vi "5492_Zero Yaw.vi"(7 "Device Number":T1, 8 "error in":errorcluster, 10 "Zero":bool) -> (0 "error out":errorcluster)   [LabVIEW 2016]
uses:
  <vilib>/Rock Robotics/WPI/ThirdParty/Sensors/navX/_TypeDefs/FRIC_navX_DeviceNumbersTypeDef.ctl
  <vilib>/Rock Robotics/WPI/ThirdParty/Sensors/navX/_TypeDefs/Z900_navX_ActionTypeDef.ctl
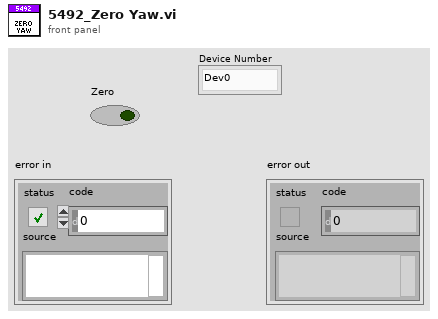
[diagram p1: front panel]
types:
  T1 = typedef "FRIC_navX_DeviceNumbersTypeDef.ctl" = enum16{"Dev0", "Dev1", "Dev2", "Dev3"}
  T2 = typedef "Z900_navX_ActionTypeDef.ctl" = enum16{"None", "Halt", "Normal Read", "Update Serial Protocol", "Update Rate Htz", "Zero-Yaw", "Zero-Displacement", "Zero-Velocity"}
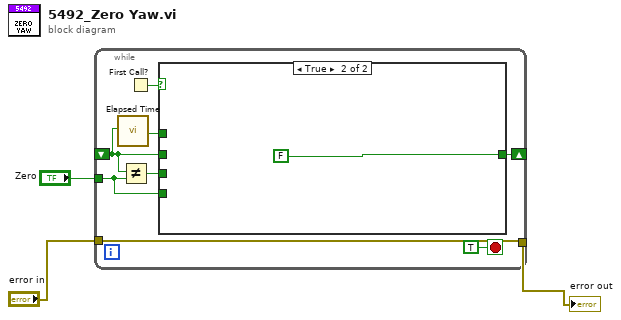
[diagram p0: block diagram]
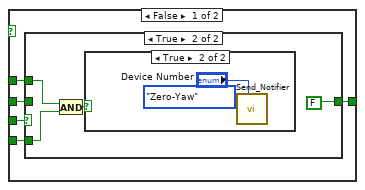
[diagram p2: hidden frame]
diagram:
  n1 = while {
    shift-right: [w10] -> _
    shift-left: _ -> [w5]
    tunnel: "Zero" -> [w7]
    tunnel: [w4] -> w2
    tunnel: "error in" -> [w4]
    stop <- TRUE stop-if-true
    n2 = call "Elapsed Time"("Reset"=w5) -> ("Time has Elapsed"=w6:bool)  [unwired: 11 in, 7 out]
    n3 = Not Equal?(x=w5, y=w7) -> (x != y?=w9:bool)
    n4 = First Call?() -> (First Call?: T/F=w8:bool)
    n5 = case shown="True" w8 {
      tunnel: [w16 FALSE] -> w10
      tunnel: w5 -> [w15 _]
      tunnel: w9 -> [w14 _]
      tunnel: w7 -> [w13 _]
      tunnel: w6 -> [w12 _]
      frame False {
        n6 = case shown="True" w14 {
          tunnel: [w17 FALSE] -> w16
          tunnel: w15 -> [w17 _]
          tunnel: w13 -> [_ w21]
          tunnel: w12 -> [_ w19]
          frame False {
          }
          frame True {
            n7 = And(x=w19, y=w21) -> (x .and. y?=w20:bool)
            n8 = case shown="True" w20 {
              frame False {
              }
              frame True {
                n9 = call <vilib>:"Send_Notifier.vi"("Device Number"="Device Number", "navX Action"=Z900_navX_ActionTypeDef."Zero-Yaw") -> ()  [unwired: 10 in]
              }
            }
          }
        }
      }
      frame True {
      }
    }
  }
  "error out" <- w2
